vi "G#Debugger_ShowAttributes.vi"(1 "VIRef":refnum<vi>, 2 "SubPanel":refnum<vi>, 3 "ClassAttributes":bool, 5 "error in (no error)":errorcluster) -> (15 "Width":i32, 19 "error out":errorcluster)   [LabVIEW 2017, in "G#Debugger.lvlib"]
uses:
  <vilib>/addons/_AddQ/G#Debugger/G#Debugger.lvlib
  <vilib>/Utility/miscctls.llb/LVPointTypeDef.ctl
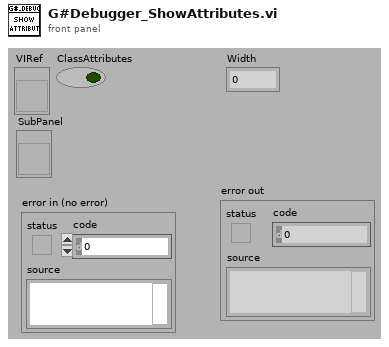
[diagram p1: front panel]
types:
  T1 = enum8{"Enabled", "Disabled", "Disabled and Grayed Out"}
  T2 = typedef "LVPointTypeDef.ctl" = cluster{"Horizontal":i16, "Vertical":i16}
  T3 = enum16{"Always On", "Always Off", "Off While Running"}
  T4 = enum32{"Invalid", "Standard", "Closed", "Hidden", "Minimized", "Maximized"}
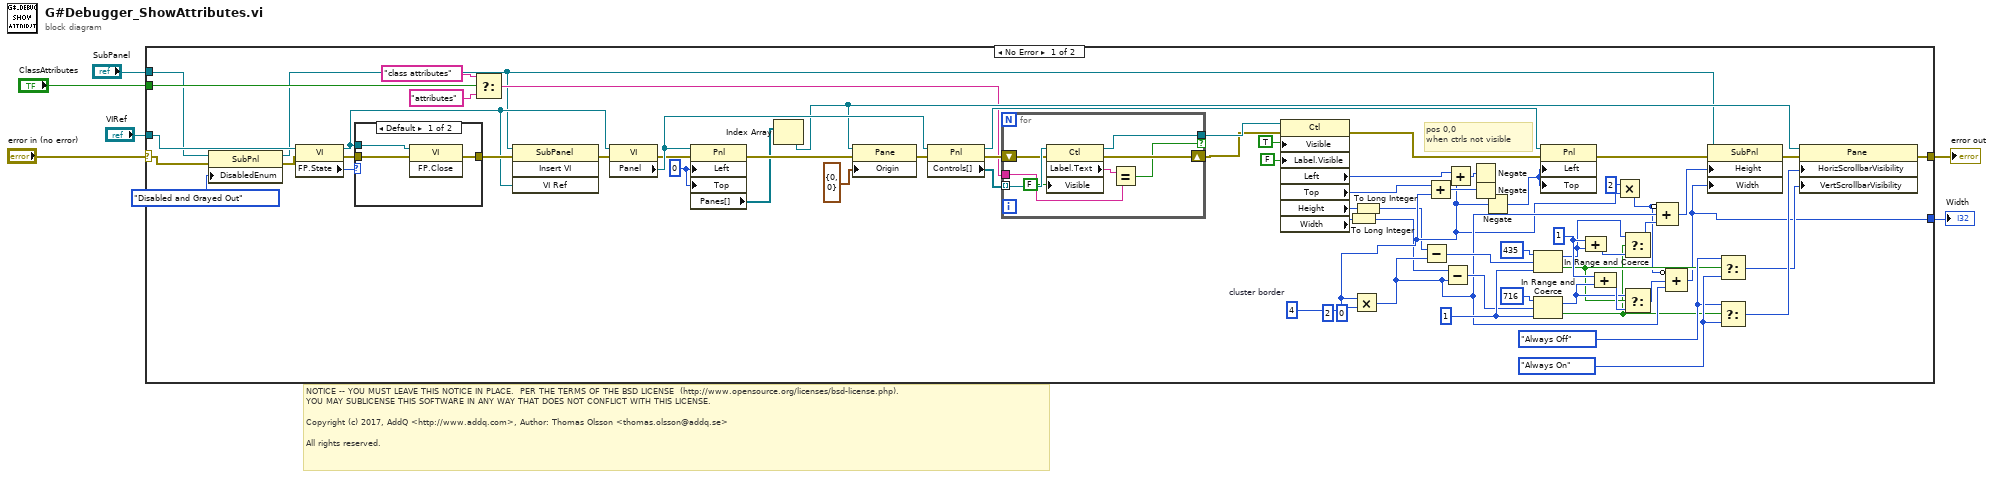
[diagram p0: block diagram]
diagram:
  # "NOTICE -- YOU MUST LEAVE THIS NOTICE IN PLACE.  PER THE TERMS OF THE BSD LICENSE  (http://www.opensource.org/licenses/bsd-license.php).\nYOU MAY SUBLICENSE THIS SOFTWARE IN ANY WAY THAT DOES NOT CONFLICT WITH THIS LICENSE.\n\nCopyright (c) 2017, AddQ <http://www.addq.com>, Author: Thomas Olsson <thomas.olsson@addq.se>\n\nAll rights reserved."
  n1 = case shown="No Error" "error in (no error)" {
    selector: "error in (no error)" -> [w41 w87]
    tunnel: [w48 w87] -> w5
    tunnel: "VIRef" -> [w52 _]
    tunnel: "ClassAttributes" -> [w51 _]
    tunnel: "SubPanel" -> [w43 _]
    tunnel: [w7 _] -> w1
    frame No Error {
      (unwired) u32 2 ("lower limit")
      w28 = 1 ("upper limit")
      w13 = 4  # cluster border
      w53 = T3."Always Off" ("Horizontal Scrollbar Visibility")
      w54 = T3."Always On" ("Horizontal Scrollbar Visibility")
      w65 = 1 ("lower limit")
      w61 = 0 ("Position:Left")
      # "pos 0,0\nwhen ctrls not visible"
      n2 = property on="Property Node" class="SubPnl"(reference=w43, error in=w41, "DisabledEnum"=T1."Disabled and Grayed Out" ("Disabled")) -> (reference out=w42:refnum<vi>, error out=w40:errorcluster)
      n3 = property class="VI"(reference=w52, error in=w40) -> (reference out=w45:refnum<vi>, error out=w72:errorcluster, "FP.State"=w74:T4)
      n4 = case shown="Default" w74 {
        tunnel: w45 -> [w85 _]
        tunnel: [w84 w86] -> w73
        tunnel: w72 -> [w83 w86]
        frame Default {
          n5 = invoke class="VI" method="FP.Close"(reference=w85, error in=w83) -> (error out=w84:errorcluster)  [unwired: 1 in, 2 out]
        }
        frame "Closed" {
        }
      }
      n6 = Select(t="class attributes" ("y"), s=w51, f="attributes" ("y")) -> (s? t:f=w50:string)
      n7 = invoke on="Invoke Node" class="SubPanel" method="Insert VI"(reference=w42, error in=w73, "VI Ref"=w45) -> (error out=w55:errorcluster)  [unwired: 1 in, 3 out]
      n8 = property class="VI"(reference=w45, error in=w55) -> (error out=w60:errorcluster, "Panel"=w69:refnum<vi>)  [unwired: 1 out]
      n9 = property class="Pnl"(reference=w69, error in=w60, "Left"=w61, "Top"=w61) -> (error out=w70:errorcluster, "Panes[]"=w66:refnum<vi>[])  [unwired: 1 out]
      n10 = Index Array(array=w66) -> (element=w67:refnum<vi>)  [unwired: 1 in]
      n11 = property class="Pane"(reference=w67, error in=w70, "Origin"=T2 {"Horizontal"=0, "Vertical"=0}) -> (error out=w71:errorcluster)  [unwired: 1 out]
      n12 = property class="Pnl"(reference=w69, error in=w71) -> (reference out=w58:refnum<vi>, error out=w57:errorcluster, "Controls[]"=w56:refnum<vi>[])
      n13 = for {
        tunnel: w56 -> [w82] mode=indexing
        tunnel: [w80] -> w22 if=w76
        shift-right: [w78] -> w21
        shift-left: w57 -> [w79]
        tunnel: w50 -> [w77]
        n14 = property class="Ctl"(reference=w82, error in=w79, "Visible"=FALSE) -> (reference out=w80:refnum<vi>, error out=w78:errorcluster, "Label.Text"=w81:string)
        n15 = Equal?(x=w81, y=w77) -> (x = y?=w76:bool)
      }
      n16 = property class="Ctl"(reference=w22, error in=w21, "Visible"=TRUE, "Label.Visible"=FALSE) -> (error out=w59:errorcluster, "Left"=w33:i32, "Top"=w39:i32, "Height"=w37:u32, "Width"=w31:u32)  [unwired: 1 out]
      n17 = To Long Integer(number=w31) -> (32bit integer=w9:i32)
      n18 = Multiply(x=w13, y=0 ("lower limit")) -> (x*y=w18:i32)
      n19 = To Long Integer(number=w37) -> (32bit integer=w10:i32)
      n20 = Subtract(x=w10, y=w18) -> (x-y=w36:i32)
      n21 = Add(x=w39, y=w13) -> (x+y=w38:i32)
      n22 = Subtract(x=w9, y=w18) -> (x-y=w30:i32)
      n23 = Add(x=w33, y=w13) -> (x+y=w32:i32)
      n24 = Negate(x=w32) -> ()  [unwired: 1 out]
      n25 = Negate(x=w38) -> ()  [unwired: 1 out]
      n26 = Negate(x=w13) -> (-x=w14:i32)
      n27 = In Range and Coerce(upper limit=435, x=w36, lower limit=w65) -> (coerced(x)=w27:i32, In Range?=w12:bool)
      n28 = In Range and Coerce(upper limit=716, x=w30, lower limit=w65) -> (coerced(x)=w24:i32, In Range?=w11:bool)
      n29 = property class="Pnl"(reference=w58, error in=w59, "Left"=w14, "Top"=w14) -> (error out=w62:errorcluster)  [unwired: 1 out]
      n30 = Compound Arithmetic op=ADD(w28, w27) -> (w26:i32)
      n31 = Compound Arithmetic op=ADD(w28, w24) -> (w25:i32)
      n32 = Multiply(x=2 ("lower limit"), y=w13) -> (x*y=w8:i32)
      n33 = Select(t=w27, s=w11, f=w26) -> (s? t:f=w17:i32)
      n34 = Select(t=w24, s=w12, f=w25) -> (s? t:f=w19:i32)
      n35 = Compound Arithmetic op=ADD(invert w8, w18, w17) -> (w16:i32)
      n36 = Compound Arithmetic op=ADD(invert w8, w19, w18) -> (w7:i32)
      n37 = property on="Property Node" class="SubPnl"(reference=w42, error in=w62, "Height"=w16, "Width"=w7) -> (error out=w49:errorcluster)  [unwired: 1 out]
      n38 = Select(t=w53, s=w12, f=w54) -> (s? t:f=w34:T3)
      n39 = Select(t=w53, s=w11, f=w54) -> (s? t:f=w35:T3)
      n40 = property class="Pane"(reference=w67, error in=w49, "HorizScrollbarVisibility"=w35, "VertScrollbarVisibility"=w34) -> (error out=w48:errorcluster)  [unwired: 1 out]
    }
    frame Error {
    }
  }
  "error out" <- w5
  "Width" <- w1
